vi "CloseManager.vi"(8 "error in (no error)":errorcluster, 11 "SequenceManager in":refnum<class "SequenceManager.lvclass">) -> (0 "error out":errorcluster, 3 "SequenceManager out":refnum<class "SequenceManager.lvclass">)   [LabVIEW 2023, in "Easy.SequenceManagerLabVIEW.lvlib" / "SequenceManager.lvclass"]
uses:
  SequenceManager.lvclass
  SequenceManager.lvclass/SequenceManager.ctl
panel:
  # "Connector Pane"
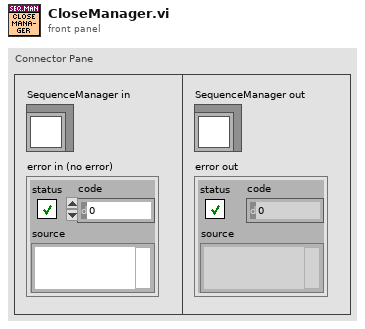
[diagram p1: front panel]
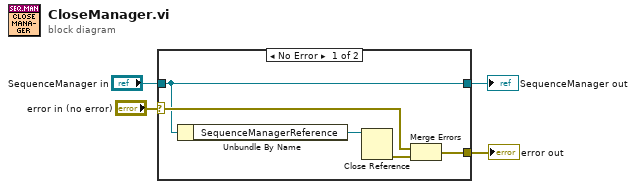
[diagram p0: block diagram]
diagram:
  n1 = case shown="No Error" "error in (no error)" {
    selector: "error in (no error)" -> [w9 w11]
    tunnel: [w7 w11] -> w3
    tunnel: [w5 w10] -> w1
    tunnel: "SequenceManager in" -> [w5 w10]
    frame No Error {
      n2 = Unbundle By Name(w5) -> ("SequenceManagerReference"=w8:refnum<k24>)
      n3 = Close Reference(reference=w8) -> (error out=w6:errorcluster)  [unwired: 1 in]
      n4 = Merge Errors(w9, w6) -> (w7:errorcluster)
    }
    frame Error {
    }
  }
  "error out" <- w3
  "SequenceManager out" <- w1
